vi "Basic End Function.vi"(8 "Error In":errorcluster) -> (0 "Error Out":errorcluster, 3 "resulting string":string)   [LabVIEW 2014]
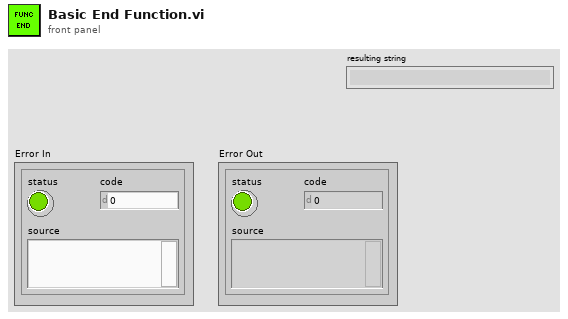
[diagram p1: front panel]
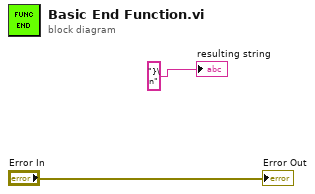
[diagram p0: block diagram]
diagram:
  "resulting string" <- "}\n" ("format string")
  "Error Out" <- "Error In"
